vi "G7_Convert_Response.vi"(7 "Response (U8)":u8[](array[numeric]) format="%x", 11 "error in (no error)":errorcluster) -> (8 "Response (string)":string, 15 "error out":errorcluster)   [LabVIEW 2020, in "G7 NFC Library.lvlib"]
uses:
  G7 NFC Library.lvlib
  <vilib>/Utility/miscctls.llb/LVDateTimeRec.ctl
panel:
  out "Sample (older)":sgl
  out "Sample (old)":sgl
  out "Sample (new)":sgl
  out "Range":u8
  out "Offset":u8
  out "Status":u8
  out "Samples (new, old, older)":u8[](array[numeric]) format="%02x"
  out "NumSamples":u8
  out "Mf":sgl
  out "unsigned byte array":u8[](array[numeric])
  out "Mo":sgl
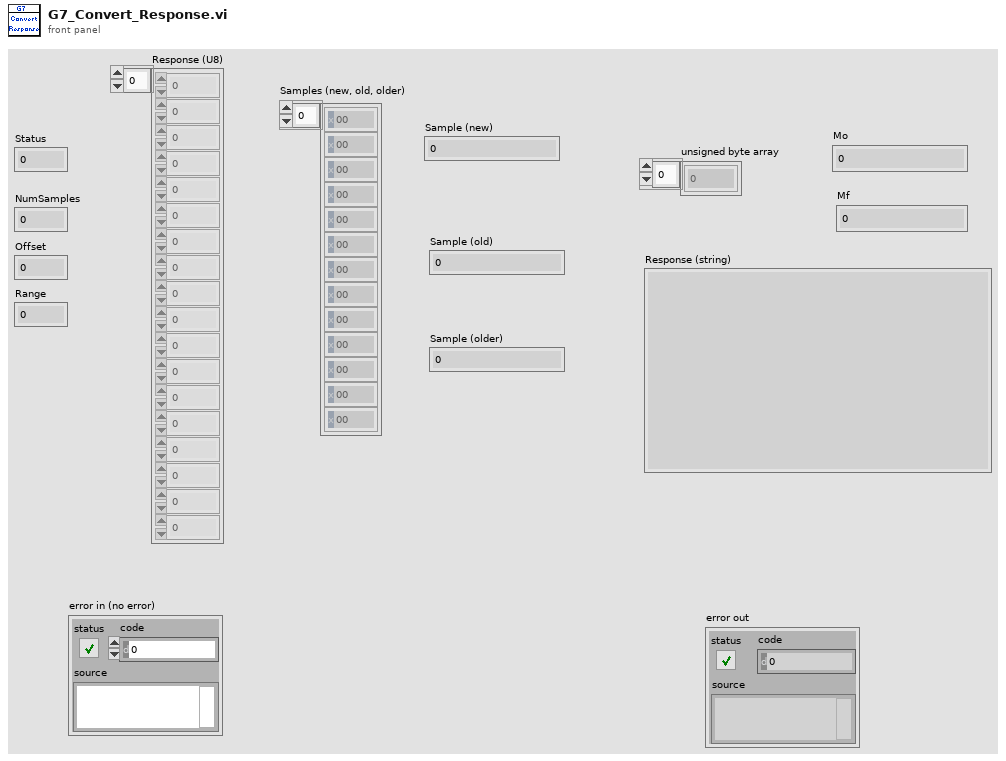
[diagram p1: front panel]
types:
  T1 = typedef "LVDateTimeRec.ctl" = cluster{"fractional second":dbl, "second":i32, "minute":i32, "hour":i32, "day of month":i32, "month":i32, "year":i32, "day of week":i32, "day of year":i32, "DST":i32}
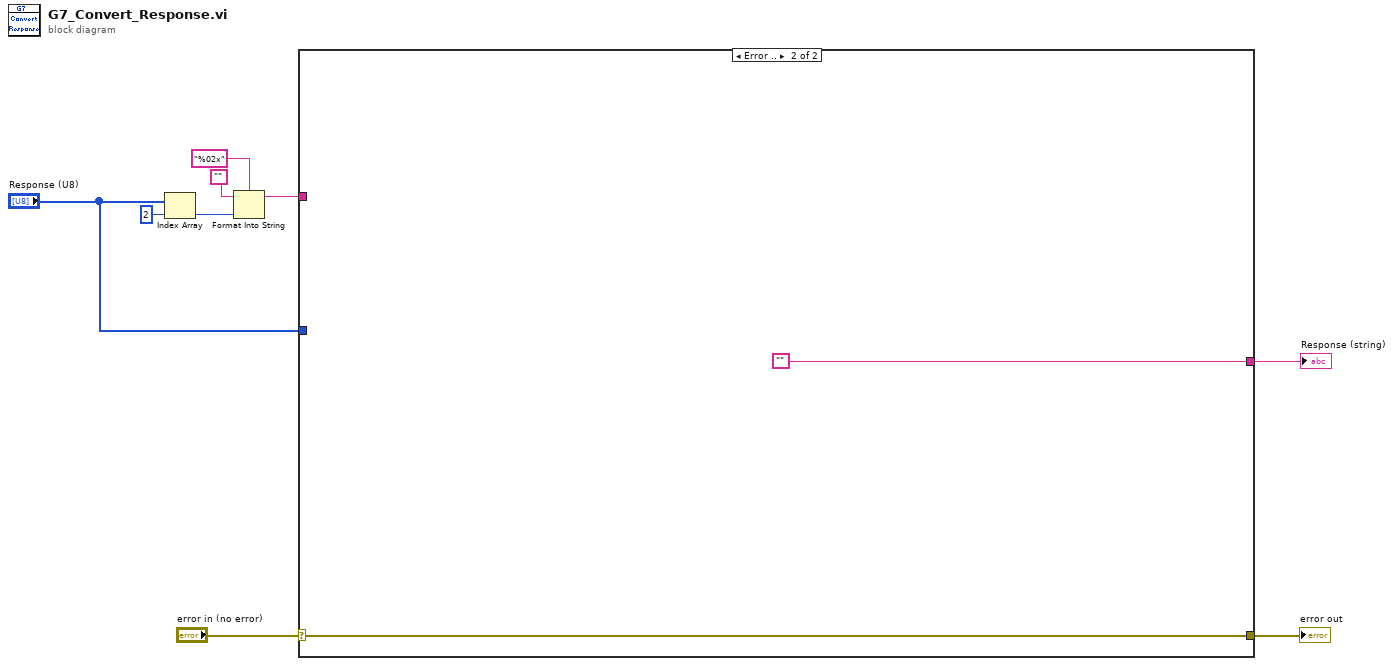
[diagram p0: block diagram]
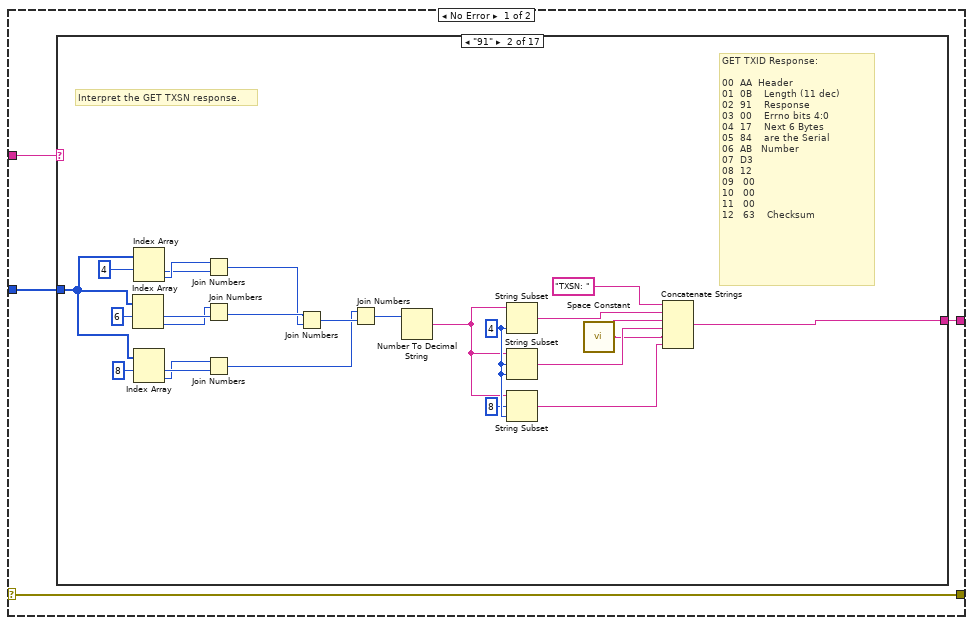
[diagram p2: hidden frame]
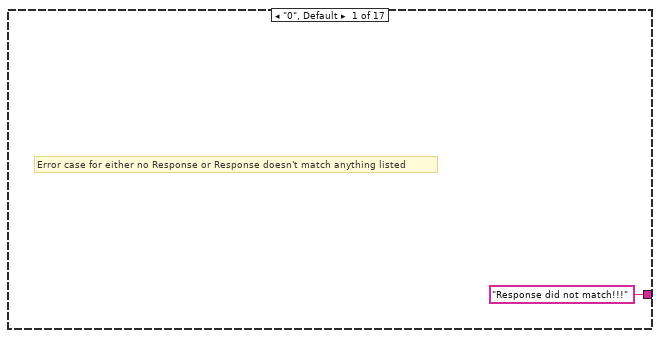
[diagram p3: hidden frame]
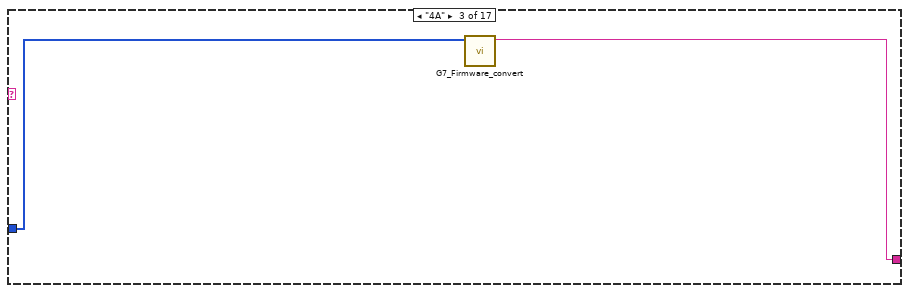
[diagram p4: hidden frame]
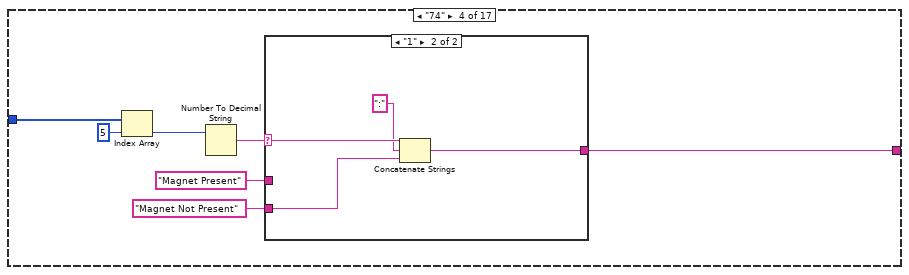
[diagram p5: hidden frame]
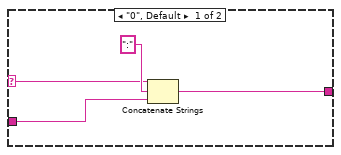
[diagram p6: hidden frame]
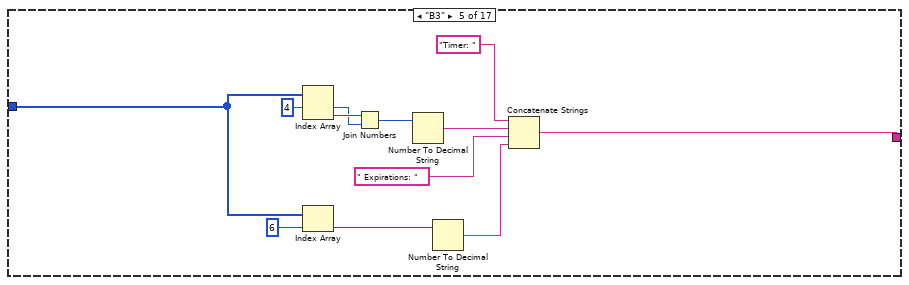
[diagram p7: hidden frame]
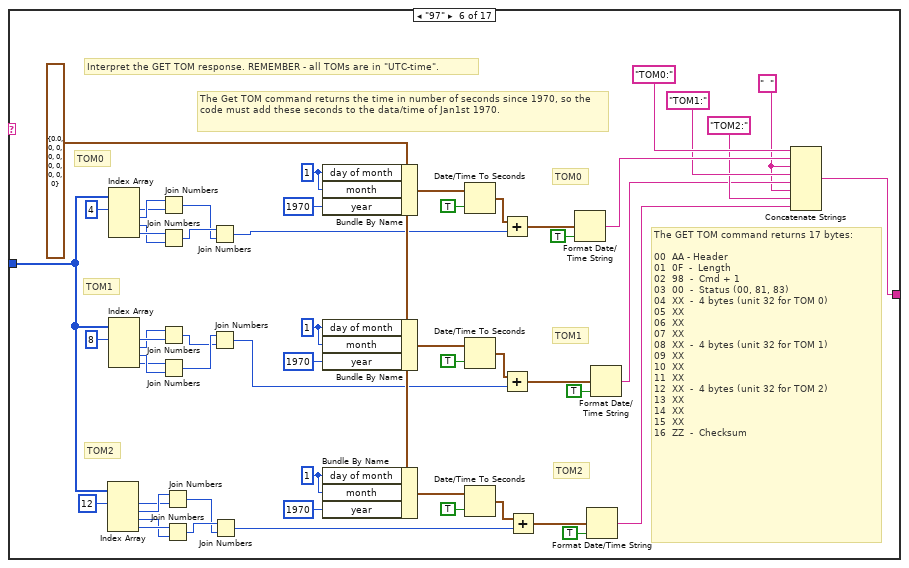
[diagram p8: hidden frame]
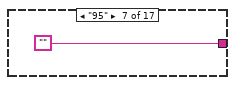
[diagram p9: hidden frame]
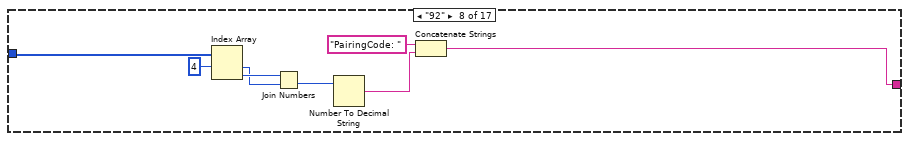
[diagram p10: hidden frame]
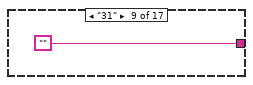
[diagram p11: hidden frame]
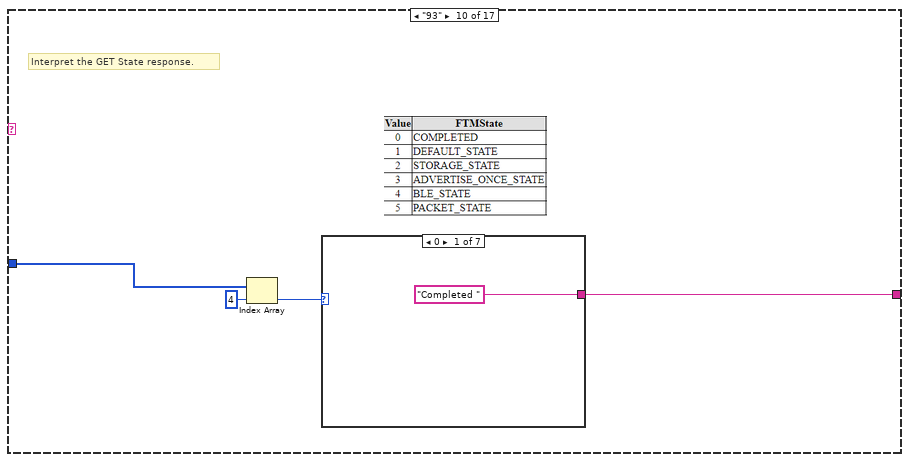
[diagram p12: hidden frame]
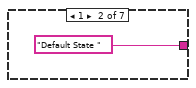
[diagram p13: hidden frame]
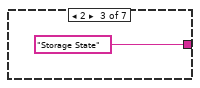
[diagram p14: hidden frame]
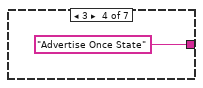
[diagram p15: hidden frame]
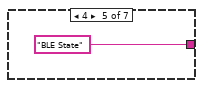
[diagram p16: hidden frame]
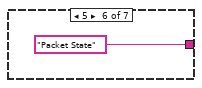
[diagram p17: hidden frame]
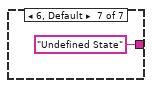
[diagram p18: hidden frame]
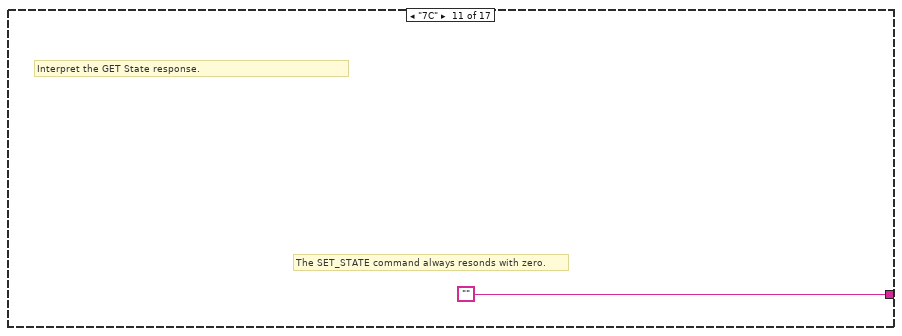
[diagram p19: hidden frame]
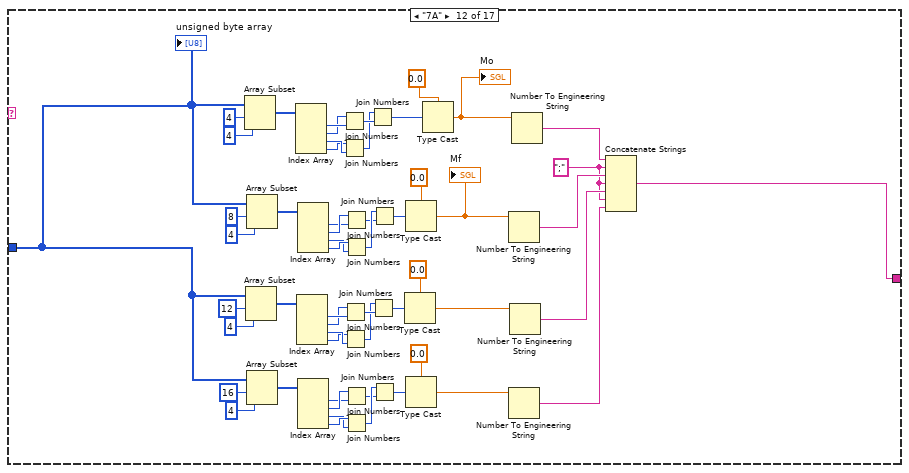
[diagram p20: hidden frame]
diagram:
  n1 = Index Array(array="Response (U8)", index=2) -> (element=w5:u8)
  n2 = Format Into String(format string="%02x", initial string="", w5) -> (resulting string=w2:string)  [unwired: 1 in, 1 out]
  n3 = case shown="Error .." "error in (no error)" {
    selector: "error in (no error)" -> [w11 w303]
    tunnel: "Response (U8)" -> [w13 _]
    tunnel: [w12 ""] -> w9
    tunnel: [w11 w303] -> w7
    tunnel: w2 -> [w10 _]
    frame No Error {
      n4 = case shown="\"91\"" w10 {
        tunnel: w13 -> [_ w32 w40 w46 w57 w75 _ w128 _ w134 _ w150 w201 w260 w280 w292 _]
        tunnel: ["Response did not match!!!" ("String") w28 w39 w41 w58 w74 "" w124 "" w133 "" w173 w200 w259 w271 w290 ""] -> w12
        frame "0", Default {
          # "Error case for either no Response or Response doesn't match anything listed"
        }
        frame "91" {
          w21 = 4 ("length (rest)")
          # "GET TXID Response:\n\n00  AA  Header\n01  0B    Length (11 dec)\n02  91    Response\n03  00    Errno bits 4:0\n04  17    Next 6 Bytes \n05  84    are the Serial\n06  AB   Number\n07  D3\n08  12\n09   00\n10   00\n11   00\n12   63    Checksum"
          # "Interpret the GET TXSN response."
          n5 = Index Array(array=w32, index #1=6 ("index")) -> (element #1=w30:u8, element #2=w29:u8)  [unwired: 1 in]
          n6 = Index Array(array=w32, index #1=4 ("index")) -> (element #1=w36:u8, element #2=w37:u8)  [unwired: 1 in]
          n7 = Index Array(array=w32, index #1=8 ("index")) -> (element #1=w33:u8, element #2=w31:u8)  [unwired: 1 in]
          n8 = Join Numbers(hi=w37, lo=w36) -> ((hi.lo)=w25:u16)
          n9 = Join Numbers(hi=w29, lo=w30) -> ((hi.lo)=w26:u16)
          n10 = Join Numbers(hi=w31, lo=w33) -> ((hi.lo)=w23:u16)
          n11 = Join Numbers(hi=w26, lo=w25) -> ((hi.lo)=w24:u32)
          n12 = Join Numbers(hi=w23, lo=w24) -> ((hi.lo)=w22:u64)
          n13 = Number To Decimal String(number=w22) -> (decimal integer string=w19:string)  [unwired: 1 in]
          n14 = String Subset(string=w19, length (rest)=w21) -> (substring=w18:string)  [unwired: 1 in]
          n15 = String Subset(string=w19, offset (0)=w21, length (rest)=w21) -> (substring=w17:string)
          n16 = String Subset(string=w19, offset (0)=8, length (rest)=w21) -> (substring=w15:string)
          n17 = call <vilib>:"Space Constant.vi"() -> ("String"=w16:string)
          n18 = Concatenate Strings("TXSN: " ("String"), w18, w16, w17, w16, w15) -> (w28:string)
        }
        frame "4A" {
          n19 = call "G7_Firmware_convert.vi"("Response (U8)"=w40) -> ("String"=w39:string)  [unwired: 10 in]
        }
        frame "74" {
          n20 = Index Array(array=w46, index=5) -> (element=w45:u8)
          n21 = Number To Decimal String(number=w45) -> (decimal integer string=w44:string)  [unwired: 1 in]
          n22 = case shown="\"1\"" w44 {
            selector: w44 -> [w50 w55]
            tunnel: "Magnet Not Present" -> [_ w53]
            tunnel: "Magnet Present" -> [w49 _]
            tunnel: [w48 w52] -> w41
            frame "0", Default {
              n23 = Concatenate Strings(w50, ":", w49) -> (w48:string)
            }
            frame "1" {
              n24 = Concatenate Strings(w55, ":", w53) -> (w52:string)
            }
          }
        }
        frame "B3" {
          n25 = Index Array(array=w57, index #1=4 ("index")) -> (element #1=w65:u8, element #2=w66:u8)  [unwired: 1 in]
          n26 = Index Array(array=w57, index=6) -> (element=w64:u8)
          n27 = Join Numbers(hi=w66, lo=w65) -> ((hi.lo)=w67:u16)
          n28 = Number To Decimal String(number=w67) -> (decimal integer string=w60:string)  [unwired: 1 in]
          n29 = Number To Decimal String(number=w64) -> (decimal integer string=w59:string)  [unwired: 1 in]
          n30 = Concatenate Strings("Timer: " ("string"), w60, " Expirations: " ("string"), w59) -> (w58:string)
        }
        frame "97" {
          w68 = "  "
          w90 = 1 ("day of month")
          w93 = 1 ("day of month")
          w100 = 1 ("day of month")
          w86 = T1 {"fractional second"=0.0, "second"=0, "minute"=0, "hour"=0, "day of month"=0, "month"=0, "year"=0, "day of week"=0, "day of year"=0, "DST"=0} ("date time rec")
          # "TOM2"
          # "TOM1"
          # "TOM0"
          # "TOM2"
          # "TOM1"
          # "TOM0"
          # "Interpret the GET TOM response. REMEMBER - all TOMs are in \"UTC-time\"."
          # "The GET TOM command returns 17 bytes:\n\n00  AA - Header\n01  0F  -  Length\n02  98  -  Cmd + 1\n03  00  -  Status (00, 81, 83)\n04  XX  -  4 bytes (unit 32 for TOM 0)\n05  XX\n06  XX\n07  XX\n08  XX  -  4 bytes (unit 32 for TOM 1)\n09  XX\n10  XX\n11  XX\n12  XX  -  4 bytes (unit 32 for TOM 2)\n13  XX\n14  XX\n15  XX\n16  ZZ  -  Checksum"
          # "The Get TOM command returns the time in number of seconds since 1970, so the code must add these seconds to the data/time of Jan1st 1970."
          n31 = Index Array(array=w75, index #1=12 ("index")) -> (element #1=w110:u8, element #2=w111:u8, element #3=w108:u8, element #4=w109:u8)  [unwired: 3 in]
          n32 = Index Array(array=w75, index #1=4 ("index")) -> (element #1=w120:u8, element #2=w121:u8, element #3=w118:u8, element #4=w119:u8)  [unwired: 3 in]
          n33 = Index Array(array=w75, index #1=8 ("index")) -> (element #1=w115:u8, element #2=w114:u8, element #3=w117:u8, element #4=w116:u8)  [unwired: 3 in]
          n34 = Join Numbers(hi=w121, lo=w120) -> ((hi.lo)=w106:u16)
          n35 = Join Numbers(hi=w119, lo=w118) -> ((hi.lo)=w107:u16)
          n36 = Join Numbers(hi=w114, lo=w115) -> ((hi.lo)=w104:u16)
          n37 = Join Numbers(hi=w116, lo=w117) -> ((hi.lo)=w105:u16)
          n38 = Join Numbers(hi=w111, lo=w110) -> ((hi.lo)=w102:u16)
          n39 = Join Numbers(hi=w109, lo=w108) -> ((hi.lo)=w103:u16)
          n40 = Join Numbers(hi=w107, lo=w106) -> ((hi.lo)=w85:u32)
          n41 = Join Numbers(hi=w105, lo=w104) -> ((hi.lo)=w84:u32)
          n42 = Join Numbers(hi=w103, lo=w102) -> ((hi.lo)=w83:u32)
          n43 = Bundle By Name(cluster=w86, "day of month"=w100, "month"=w100, "year"=1970) -> (w101:T1)
          n44 = Bundle By Name(cluster=w86, "day of month"=w93, "month"=w93, "year"=1970) -> (w92:T1)
          n45 = Bundle By Name(cluster=w86, "day of month"=w90, "month"=w90, "year"=1970) -> (w91:T1)
          n46 = Date/Time To Seconds(1:TRUE ("is UTC (F)"), 2:w101) -> (0:w97:timestamp)
          n47 = Date/Time To Seconds(1:TRUE ("is UTC (F)"), 2:w92) -> (0:w96:timestamp)
          n48 = Date/Time To Seconds(1:TRUE ("is UTC (F)"), 2:w91) -> (0:w87:timestamp)
          n49 = Add(x=w97, y=w85) -> (x+y=w77:timestamp)
          n50 = Add(x=w96, y=w84) -> (x+y=w78:timestamp)
          n51 = Add(x=w87, y=w83) -> (x+y=w82:timestamp)
          n52 = Format Date/Time String(seconds (now)=w77, UTC format=TRUE) -> (date/time string=w76:string)  [unwired: 1 in]
          n53 = Format Date/Time String(seconds (now)=w82, UTC format=TRUE) -> (date/time string=w71:string)  [unwired: 1 in]
          n54 = Format Date/Time String(seconds (now)=w78, UTC format=TRUE) -> (date/time string=w69:string)  [unwired: 1 in]
          n55 = Concatenate Strings("TOM0:", w76, w68, "TOM1:", w69, w68, "TOM2:", w71) -> (w74:string)
        }
        frame "95" {
        }
        frame "92" {
          n56 = Index Array(array=w128, index #1=4 ("index")) -> (element #1=w130:u8, element #2=w131:u8)  [unwired: 1 in]
          n57 = Join Numbers(hi=w131, lo=w130) -> ((hi.lo)=w127:u16)
          n58 = Number To Decimal String(number=w127) -> (decimal integer string=w126:string)  [unwired: 1 in]
          n59 = Concatenate Strings("PairingCode: " ("string"), w126) -> (w124:string)
        }
        frame "31" {
        }
        frame "93" {
          # "Interpret the GET State response."
          n60 = Index Array(array=w134, index=4) -> (element=w135:u8)
          n61 = case shown="0" w135 {
            tunnel: ["Completed " "Default State " "Storage State" "Advertise Once State" "BLE State" "Packet State" "Undefined State"] -> w133
            frame 0 {
            }
            frame 1 {
            }
            frame 2 {
            }
            frame 3 {
            }
            frame 4 {
            }
            frame 5 {
            }
            frame 6, Default {
            }
          }
        }
        frame "7C" {
          # "The SET_STATE command always resonds with zero."
          # "Interpret the GET State response."
        }
        frame "7A" {
          w146 = ";"
          n62 = Array Subset(array=w150, index=4, length=4) -> (w189:u8[])
          n63 = Array Subset(array=w150, index=12, length=4) -> (w162:u8[])
          n64 = Array Subset(array=w150, index=8, length=4) -> (w187:u8[])
          n65 = Array Subset(array=w150, index=16, length=4) -> (w161:u8[])
          n66 = Index Array(array=w189) -> (element #1=w197:u8, element #2=w196:u8, element #3=w195:u8, element #4=w194:u8)  [unwired: 4 in]
          n67 = Index Array(array=w162) -> (element #1=w170:u8, element #2=w169:u8, element #3=w168:u8, element #4=w167:u8)  [unwired: 4 in]
          n68 = Index Array(array=w187) -> (element #1=w179:u8, element #2=w180:u8, element #3=w181:u8, element #4=w182:u8)  [unwired: 4 in]
          n69 = Index Array(array=w161) -> (element #1=w153:u8, element #2=w154:u8, element #3=w155:u8, element #4=w156:u8)  [unwired: 4 in]
          n70 = Join Numbers(hi=w196, lo=w197) -> ((hi.lo)=w193:u16)
          n71 = Join Numbers(hi=w194, lo=w195) -> ((hi.lo)=w192:u16)
          n72 = Join Numbers(hi=w169, lo=w170) -> ((hi.lo)=w166:u16)
          n73 = Join Numbers(hi=w167, lo=w168) -> ((hi.lo)=w165:u16)
          n74 = Join Numbers(hi=w180, lo=w179) -> ((hi.lo)=w183:u16)
          n75 = Join Numbers(hi=w182, lo=w181) -> ((hi.lo)=w184:u16)
          n76 = Join Numbers(hi=w154, lo=w153) -> ((hi.lo)=w157:u16)
          n77 = Join Numbers(hi=w156, lo=w155) -> ((hi.lo)=w158:u16)
          n78 = Join Numbers(hi=w192, lo=w193) -> ((hi.lo)=w191:u32)
          n79 = Join Numbers(hi=w165, lo=w166) -> ((hi.lo)=w164:u32)
          n80 = Join Numbers(hi=w184, lo=w183) -> ((hi.lo)=w185:u32)
          n81 = Join Numbers(hi=w158, lo=w157) -> ((hi.lo)=w159:u32)
          n82 = Type Cast(type=sgl 0.0, x=w164) -> (*(type *) &x=w149:sgl)
          n83 = Type Cast(type=sgl 0.0, x=w185) -> (*(type *) &x=w176:sgl)
          "Mf" <- w176
          n84 = Type Cast(type=sgl 0.0, x=w159) -> (*(type *) &x=w148:sgl)
          n85 = Type Cast(type=sgl 0.0, x=w191) -> (*(type *) &x=w188:sgl)
          "Mo" <- w188
          n86 = Number To Engineering String(4:w176) -> (0:w174:string)  [unwired: 3 in]
          n87 = Number To Engineering String(4:w148) -> (0:w145:string)  [unwired: 3 in]
          n88 = Number To Engineering String(4:w149) -> (0:w147:string)  [unwired: 3 in]
          n89 = Number To Engineering String(4:w188) -> (0:w175:string)  [unwired: 3 in]
          n90 = Concatenate Strings(w175, w146, w174, w146, w147, w146, w145) -> (w173:string)
          "unsigned byte array" <- w150
        }
        frame "7E" {
          w205 = ";"
          w253 = 8 ("index")
          n91 = Array Size(array=w201) -> (size(s)=w254:i32)
          n92 = Add(x=w253, y=1) -> (x+y=w251:i32)
          n93 = Index Array(array=w201, index #1=4 ("index"), index #2=5 ("index"), index #3=6 ("index"), index #4=7 ("index")) -> (element #1=→"Status":u8, element #2=→"NumSamples":u8, element #3=→"Offset":u8, element #4=→"Range":u8)
          n94 = Subtract(x=w254, y=w251) -> (x-y=w250:i32)
          n95 = Array Subset(array=w201, index=w253, length=w250) -> (w211:u8[])
          "Samples (new, old, older)" <- w211
          n96 = Array Subset(array=w211, index=8, length=4) -> (w212:u8[])
          n97 = Array Subset(array=w211, index=4, length=4) -> (w233:u8[])
          n98 = Array Subset(array=w211, index=0, length=4) -> (w234:u8[])
          n99 = Index Array(array=w212) -> (element #1=w220:u8, element #2=w219:u8, element #3=w218:u8, element #4=w217:u8)  [unwired: 4 in]
          n100 = Index Array(array=w233) -> (element #1=w225:u8, element #2=w226:u8, element #3=w227:u8, element #4=w228:u8)  [unwired: 4 in]
          n101 = Index Array(array=w234) -> (element #1=w242:u8, element #2=w241:u8, element #3=w240:u8, element #4=w239:u8)  [unwired: 4 in]
          n102 = Join Numbers(hi=w219, lo=w220) -> ((hi.lo)=w216:u16)
          n103 = Join Numbers(hi=w217, lo=w218) -> ((hi.lo)=w215:u16)
          n104 = Join Numbers(hi=w226, lo=w225) -> ((hi.lo)=w229:u16)
          n105 = Join Numbers(hi=w228, lo=w227) -> ((hi.lo)=w230:u16)
          n106 = Join Numbers(hi=w241, lo=w242) -> ((hi.lo)=w238:u16)
          n107 = Join Numbers(hi=w239, lo=w240) -> ((hi.lo)=w237:u16)
          n108 = Join Numbers(hi=w215, lo=w216) -> ((hi.lo)=w214:u32)
          n109 = Join Numbers(hi=w230, lo=w229) -> ((hi.lo)=w231:u32)
          n110 = Join Numbers(hi=w237, lo=w238) -> ((hi.lo)=w236:u32)
          n111 = Type Cast(type=sgl 0.0, x=w214) -> (*(type *) &x=w206:sgl)
          "Sample (older)" <- w206
          n112 = Type Cast(type=sgl 0.0, x=w231) -> (*(type *) &x=w207:sgl)
          "Sample (old)" <- w207
          n113 = Type Cast(type=sgl 0.0, x=w236) -> (*(type *) &x=w208:sgl)
          "Sample (new)" <- w208
          n114 = Number To Engineering String(4:w208) -> (0:w204:string)  [unwired: 3 in]
          n115 = Number To Engineering String(4:w206) -> (0:w202:string)  [unwired: 3 in]
          n116 = Number To Engineering String(4:w207) -> (0:w203:string)  [unwired: 3 in]
          n117 = Concatenate Strings(w204, w205, w203, w205, w202) -> (w200:string)
        }
        frame "22" {
          # "Interpret the GET Battery Voltages response."
          # "Voltages: Satatic, Dynamic"
          n118 = Index Array(array=w260, index #1=4 ("index")) -> (element #1=w268:u8, element #2=w267:u8)  [unwired: 1 in]
          n119 = Index Array(array=w260, index #1=6 ("index")) -> (element #1=w270:u8, element #2=w269:u8)  [unwired: 1 in]
          n120 = Join Numbers(hi=w267, lo=w268) -> ((hi.lo)=w264:u16)
          n121 = Join Numbers(hi=w269, lo=w270) -> ((hi.lo)=w263:u16)
          n122 = Number To Decimal String(number=w264) -> (decimal integer string=w262:string)  [unwired: 1 in]
          n123 = Number To Decimal String(number=w263) -> (decimal integer string=w257:string)  [unwired: 1 in]
          n124 = Concatenate Strings("Static:" ("string"), w262, "  ", "Dynamic:" ("string"), w257) -> (w259:string)
        }
        frame "C2" {
          # "Interpret the GET Temperature response."
          # "This is a bitmask of enabled and detected temperature sensors."
          # "Get Temp Response Format:\n\nAA  -  Header\n08    -  Length \nC3   -  Response (C2+1)\n00   -  Tx Status\n57    -  Bit-masked Temp Status (57 desired)\nD0   -  centi-degrees C (4 bytes) unit 32\n08\n00\n00 \n44   -  Checksum"
          # "Temp"
          # "Status (should be 0x57)"
          n125 = Index Array(array=w280, index #1=4 ("index")) -> (element #1=w277:u8, element #2=w279:u8, element #3=w286:u8)  [unwired: 2 in]
          n126 = Join Numbers(hi=w286, lo=w279) -> ((hi.lo)=w284:u16)
          n127 = Divide(x=w284, y=u16 100) -> (x/y=w282:dbl)
          n128 = Format Into String(format string="%02x", w277) -> (resulting string=w273:string)  [unwired: 2 in, 1 out]
          n129 = Number To Fractional String(number=w282, precision (6)=i16 2) -> (F-format string=w276:string)  [unwired: 2 in]
          n130 = Concatenate Strings("Temp:" ("string"), w276, "   ", "Status:" ("string"), w273) -> (w271:string)
        }
        frame "56" {
          # "Interpret the GET Battery Type response."
          n131 = Index Array(array=w292, index=6) -> (element=w289:u8)
          n132 = Number To Decimal String(number=w289) -> (decimal integer string=w288:string)  [unwired: 1 in]
          n133 = case shown="\"0\", Default" w288 {
            tunnel: ["Panasonic" "Murata" "Invalid" "Invalid" "Maxell" "Invalid" "Invalid"] -> w287
            frame "5" {
            }
            frame "6" {
            }
            frame "0", Default {
            }
            frame "1" {
            }
            frame "2" {
            }
            frame "3" {
            }
            frame "4" {
            }
          }
          n134 = Concatenate Strings("Type:", w287) -> (w290:string)
        }
        frame "4D" {
          # "The SET_STATE command has no response text."
          # "0x4E: Convert the Switch from CGM to FTM Mode (0x4D) Response"
        }
      }
    }
    frame Error {
    }
  }
  "Response (string)" <- w9
  "error out" <- w7
